vi "SAOMM-Initialize.vi"() -> ()   [LabVIEW 2011]
panel:
  in  "Bool Refnum":refnum<vi>
  out "PRAMMS Error OUT":errorcluster
  out "PRAMMS-COMM OUT":refnum<visa-resource-name>="COM4"
  in  "PRAMMS Error IN":errorcluster
  in  "PRAMMS-COMM IN":refnum<visa-resource-name>="COM4"
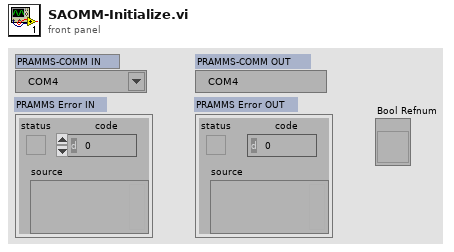
[diagram p1: front panel]
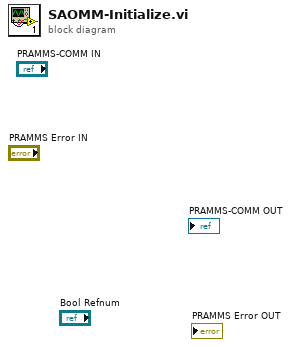
[diagram p0: block diagram]
diagram:
